vi "InstrChoice2.vi"(0 "Bras_OUT":bool, 5 "instruments.ini":path=path "C:/BonOMM_git/Config/instruments.ini") -> (6 "This VI's Path":path, 10 "Instrument Primaire OUT":string, 12 "Instrument Secondaire OUT":string, 14 "Instrument OUT":string, 15 "FoV 3":dbl caption="Champ de Vue" format="%.2g", 16 "foynom 3":i32 caption="Foyer nominale à 0°", 17 "atherm 3":dbl caption="Coefficient d'athermalisation" format="%.3g", 18 "exclusion 3":path caption="Chemin vers le fichier d'exclusion", 19 "collim 3":path caption="Chemin vers le fichier de collimation")   [LabVIEW 2019]
uses:
  <vilib>/Utility/config.llb/Read Key (String).vi
  <vilib>/Utility/config.llb/Read Key (Double).vi
  <vilib>/Utility/config.llb/Read Key (I32).vi
  <vilib>/Utility/config.llb/Read Key (Path).vi
  <vilib>/Utility/config.llb/Write Key (String).vi
  <vilib>/Utility/config.llb/Write Key (Boolean).vi
  <vilib>/Utility/config.llb/NI_LVConfig.lvlib
panel:
  out "Bool_primaire":bool
  out "Bool-Secondaire":bool
  out "Instrument Secondaire  IN":string
  out "Instrument Primaire  IN":string
  out "collim 2":path caption="Chemin vers le fichier de collimation"
  out "exclusion 2":path caption="Chemin vers le fichier d'exclusion"
  out "atherm 2":dbl caption="Coefficient d'athermalisation" format="%.3g"
  out "foynom 2":i32 caption="Foyer nominale à 0°"
  out "FoV 2":dbl caption="Champ de Vue" format="%.2g"
  in  "Instrument secondaire":i32(ring) items=["Pesto", "POMM", "CPAPIR", "Simon", "Spectro", "SpiOMM", "PANO-II+CCD4Kx4K", "CCD4Kx4K", "PANO-I+EMCCD", "POLARIMETRE"]
  out "collim":path caption="Chemin vers le fichier de collimation"
  out "exclusion":path caption="Chemin vers le fichier d'exclusion"
  out "FoV":dbl caption="Champ de Vue" format="%.2g"
  out "atherm":dbl caption="Coefficient d'athermalisation" format="%.3g"
  out "foynom":i32 caption="Foyer nominale à 0°"
  in  "ok":bool
  in  "Instruments primaire":i32(ring) items=["Pesto", "POMM", "CPAPIR", "Simon", "Spectro", "SpiOMM", "PANO-II+CCD4Kx4K", "CCD4Kx4K", "PANO-I+EMCCD", "POLARIMETRE"]
  # "[minutes d'arc]"
  # "[minutes d'arc]"
  # "[ADU]"
  # "[ADU]"
  # "[ADU/°K]"
  # "[ADU/°K]"
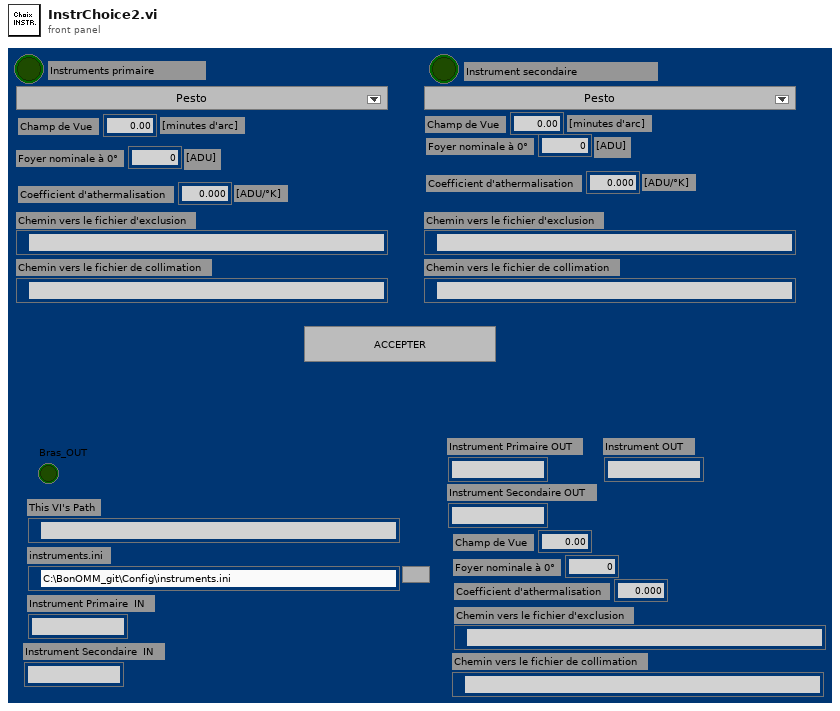
[diagram p1: front panel]
types:
  T1 = typedef "NI_LVConfig.lvlib/Config Data RefNum.ctl" = refnum<k1>
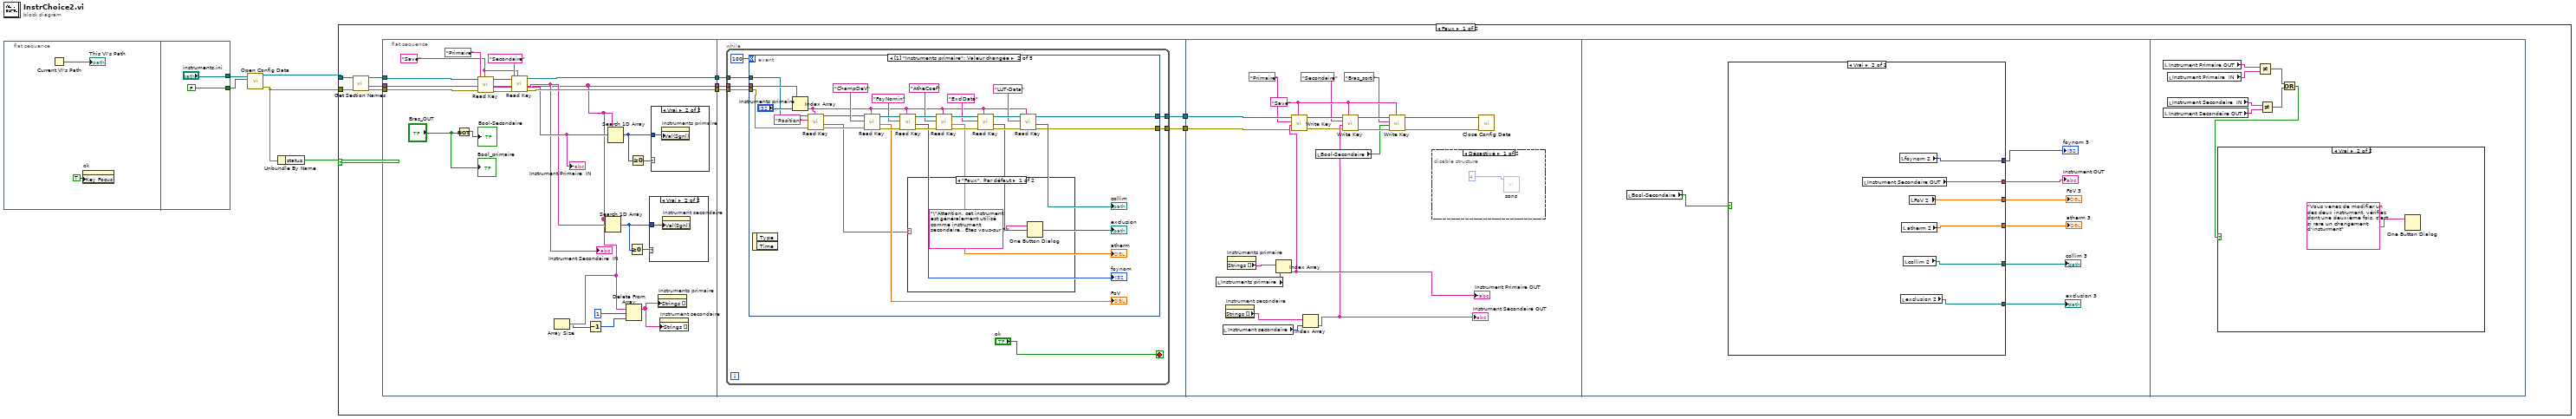
[diagram p0: block diagram]
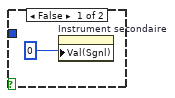
[diagram p2: hidden frame]
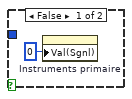
[diagram p3: hidden frame]
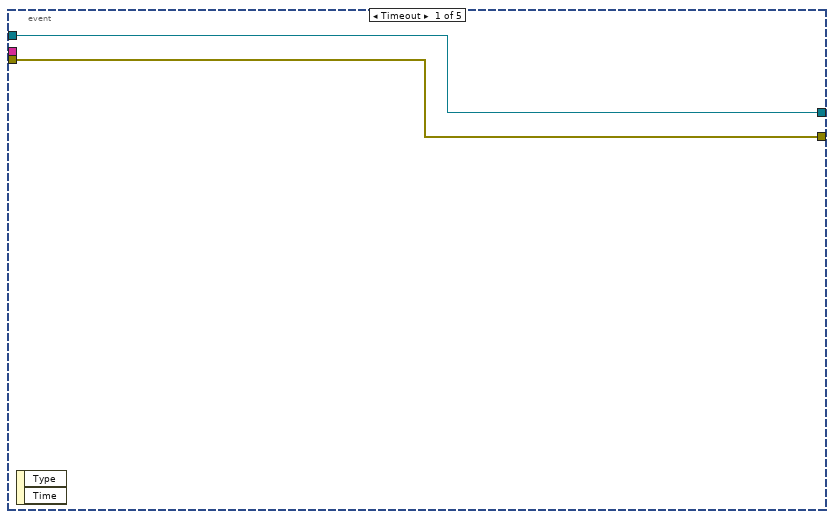
[diagram p4: hidden frame]
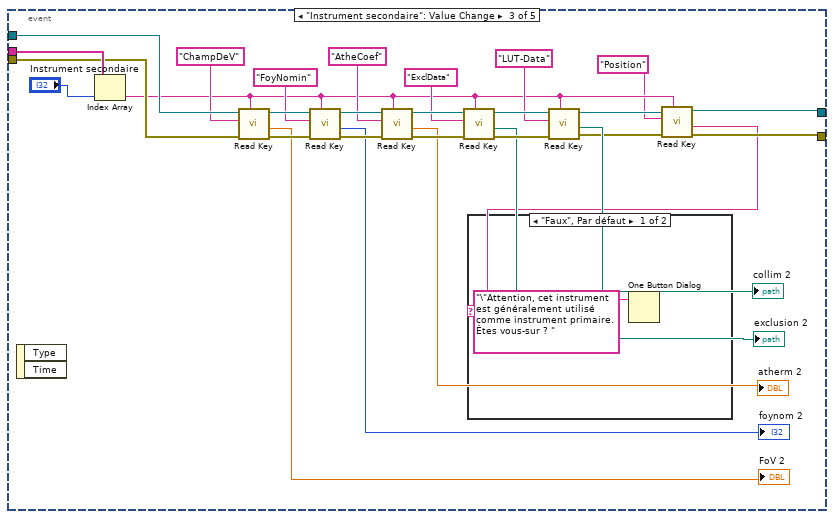
[diagram p6: hidden frame]
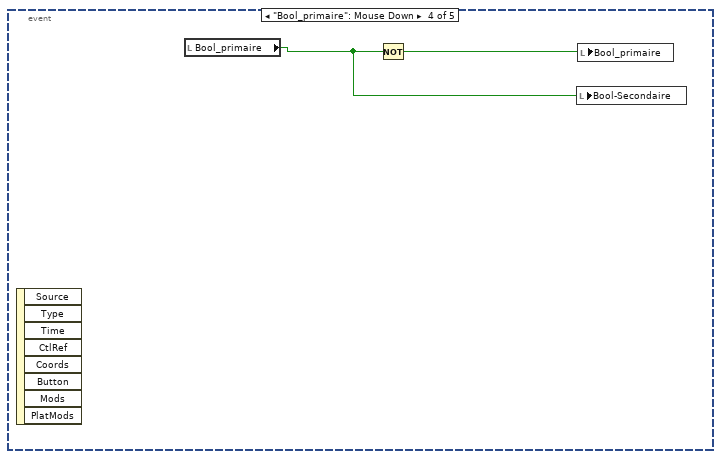
[diagram p8: hidden frame]
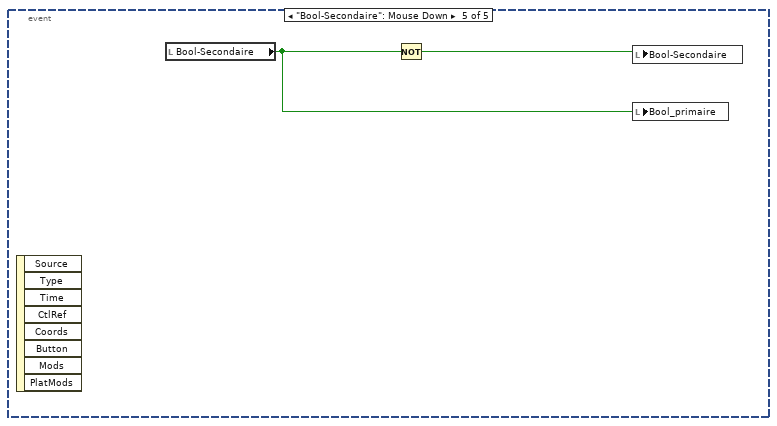
[diagram p9: hidden frame]
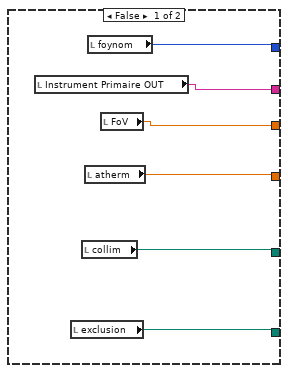
[diagram p11: hidden frame]
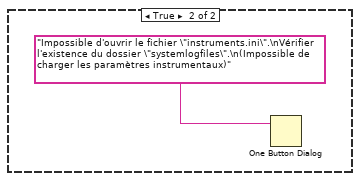
[diagram p13: hidden frame]
diagram:
  n1 = flat-sequence {
    tunnel: [FALSE ("create file if necessary (T)")] -> w5
    tunnel: ["instruments.ini"] -> w1
    frame #0 {
      n2 = Current VI's Path() -> (path=→"This VI's Path":path)
      n3 = property on="ok" class="Bool"("Key Focus"=TRUE) -> ()  [unwired: 2 in, 2 out]
    }
    frame #1 {
    }
  }
  n4 = call <vilib>:"Open Config Data.vi"("create file if necessary (T)"=w5, "configuration file path"=w1) -> ("error out"=w3:errorcluster, "refnum"=w4:T1)  [unwired: 7 in, 1 out]
  n5 = Unbundle By Name(w3) -> ("status"=w2:bool)
  n6 = case shown="Faux" w2 {
    tunnel: w4 -> [w19 _]
    tunnel: w3 -> [w18 _]
    frame False {
      n7 = call <vilib>:"Get Section Names.vi"("error in (no error)"=w18, "refnum"=w19) -> ("error out"=w15:errorcluster, "section names"=w16:string[], "refnum out"=w17:T1)  [unwired: 7 in]
      n8 = flat-sequence {
        tunnel: w17 -> [w23]
        tunnel: w16 -> [w27]
        tunnel: [w34] -> w14
        tunnel: w15 -> [w22]
        tunnel: [w37] -> w13
        tunnel: [w27] -> w12
        tunnel: w14 -> [w48]
        tunnel: w13 -> [w49]
        tunnel: w12 -> [w50]
        tunnel: [w47] -> w11
        tunnel: [w46] -> w10
        tunnel: w11 -> [w141]
        tunnel: w10 -> [w140]
        frame #0 {
          w24 = "Save" ("section")
          n9 = Not(x="Bras_OUT") -> (.not. x?=→"Bool-Secondaire":bool)
          n10 = call-poly <vilib>:"Read Key.vi"("section"=w24, "error in (no error)"=w22, "key"="Primaire", "refnum"=w23) -> ("error out"=w35:errorcluster, "value"=w33:string, "refnum out"=w38:T1)  [unwired: 4 in, 1 out]
          "Instrument Primaire  IN" <- w33
          n11 = call-poly <vilib>:"Read Key.vi"("section"=w24, "error in (no error)"=w35, "key"="Secondaire", "refnum"=w38) -> ("error out"=w34:errorcluster, "value"=w30:string, "refnum out"=w37:T1)  [unwired: 4 in, 1 out]
          "Instrument Secondaire  IN" <- w30
          n12 = Array Size(array=w27) -> (size(s)=w25:i32)
          n13 = Decrement(x=w25) -> (x-1=w26:i32)
          n14 = Search 1D Array(1D array=w27, element=w30) -> (index of element=w31:i32)  [unwired: 1 in]
          n15 = Search 1D Array(1D array=w27, element=w33) -> (index of element=w40:i32)  [unwired: 1 in]
          n16 = Delete From Array(array=w27, length=1 ("longueur"), index=w26) -> (array with subset deleted=w28:string[])  [unwired: 1 out]
          n17 = Greater Or Equal To 0?(x=w31) -> (x >= 0?=w32:bool)
          n18 = Greater Or Equal To 0?(x=w40) -> (x >= 0?=w41:bool)
          n19 = case shown="Vrai" w32 {
            tunnel: w31 -> [_ w43]
            frame False {
              n20 = property on="Instrument secondaire" class="MDér (strict)"("Val(Sgnl)"=0) -> ()  [unwired: 2 in, 2 out]
            }
            frame True {
              n21 = property on="Instrument secondaire" class="MDér (strict)"("Val(Sgnl)"=w43) -> ()  [unwired: 2 in, 2 out]
            }
          }
          n22 = case shown="Vrai" w41 {
            tunnel: w40 -> [_ w45]
            frame False {
              n23 = property on="Instruments primaire" class="MDér (strict)"("Val(Sgnl)"=0) -> ()  [unwired: 2 in, 2 out]
            }
            frame True {
              n24 = property on="Instruments primaire" class="MDér (strict)"("Val(Sgnl)"=w45) -> ()  [unwired: 2 in, 2 out]
            }
          }
          n25 = property on="Instruments primaire" class="MDér (strict)"("Strings []"=w28) -> ()  [unwired: 2 in, 2 out]
          n26 = property on="Instrument secondaire" class="MDér (strict)"("Strings []"=w28) -> ()  [unwired: 2 in, 2 out]
          "Bool_primaire" <- "Bras_OUT"
        }
        frame #1 {
          n27 = while {
            tunnel: w50 -> [w57]
            tunnel: w49 -> [w56]
            tunnel: w48 -> [w55]
            tunnel: [w53] -> w47
            tunnel: [w52] -> w46
            stop <- "ok" stop-if-true
            n28 = event shown="[1] \"Instruments primaire\": Valeur changée" {
              selector: _ -> [_ _ _ _ _]
              dyn-events: _ -> [_ _ _ _ _]
              timeout: 100 ("milliseconds to wait") -> [_ _ _ _ _]
              tunnel: w57 -> [_ w87 w118 _ _]
              tunnel: w56 -> [w59 w63 w117 _ _]
              tunnel: w55 -> [w58 w62 w116 _ _]
              tunnel: [w59 w68 w93 _ _] -> w53
              tunnel: [w58 w67 w94 _ _] -> w52
              event Timeout {
                n29 = event-data() -> ()  [unwired: 1 in, 2 out]
              }
              event "Instruments primaire": Value Change {
                n30 = event-data() -> ()  [unwired: 1 in, 2 out]
                n31 = Index Array(array=w87, index="Instruments primaire") -> (element=w65:string)
                n32 = call-poly <vilib>:"Read Key.vi"("section"=w65, "error in (no error)"=w62, "key"="Position", "refnum"=w63) -> ("error out"=w64:errorcluster, "value"=w60:string, "refnum out"=w66:T1)  [unwired: 4 in, 1 out]
                n33 = call-poly <vilib>:"Read Key.vi"("section"=w65, "error in (no error)"=w64, "key"="ChampDeV", "refnum"=w66) -> ("error out"=w85:errorcluster, "value"=→"FoV":dbl, "refnum out"=w86:T1)  [unwired: 4 in, 1 out]
                n34 = call-poly <vilib>:"Read Key.vi"("section"=w65, "error in (no error)"=w85, "key"="FoyNomin", "refnum"=w86) -> ("error out"=w83:errorcluster, "value"=→"foynom":i32, "refnum out"=w84:T1)  [unwired: 4 in, 1 out]
                n35 = case shown="\"Faux\", Par défaut" w60 {
                  frame "Faux", Default {
                    n36 = One Button Dialog(message="\"Attention, cet instrument est généralement utilisé comme instrument secondaire,. Êtes vous-sur ? ") -> ()  [unwired: 1 in, 1 out]
                  }
                  frame "Primaire" {
                  }
                }
                n37 = call-poly <vilib>:"Read Key.vi"("section"=w65, "error in (no error)"=w83, "key"="AtheCoef", "refnum"=w84) -> ("error out"=w79:errorcluster, "value"=→"atherm":dbl, "refnum out"=w80:T1)  [unwired: 4 in, 1 out]
                n38 = call-poly <vilib>:"Read Key.vi"("section"=w65, "error in (no error)"=w79, "key"="ExclData", "refnum"=w80) -> ("error out"=w82:errorcluster, "value"=→"exclusion":path, "refnum out"=w81:T1)  [unwired: 4 in, 1 out]
                n39 = call-poly <vilib>:"Read Key.vi"("section"=w65, "error in (no error)"=w82, "key"="LUT-Data", "refnum"=w81) -> ("error out"=w67:errorcluster, "value"=→"collim":path, "refnum out"=w68:T1)  [unwired: 4 in, 1 out]
              }
              event "Instrument secondaire": Value Change {
                n40 = event-data() -> ()  [unwired: 1 in, 2 out]
                n41 = Index Array(array=w118, index="Instrument secondaire") -> (element=w92:string)
                n42 = call-poly <vilib>:"Read Key.vi"("section"=w92, "error in (no error)"=w116, "key"="ChampDeV", "refnum"=w117) -> ("error out"=w114:errorcluster, "value"=→"FoV 2":dbl, "refnum out"=w115:T1)  [unwired: 4 in, 1 out]
                n43 = call-poly <vilib>:"Read Key.vi"("section"=w92, "error in (no error)"=w114, "key"="FoyNomin", "refnum"=w115) -> ("error out"=w112:errorcluster, "value"=→"foynom 2":i32, "refnum out"=w113:T1)  [unwired: 4 in, 1 out]
                n44 = call-poly <vilib>:"Read Key.vi"("section"=w92, "error in (no error)"=w112, "key"="AtheCoef", "refnum"=w113) -> ("error out"=w108:errorcluster, "value"=→"atherm 2":dbl, "refnum out"=w109:T1)  [unwired: 4 in, 1 out]
                n45 = call-poly <vilib>:"Read Key.vi"("section"=w92, "error in (no error)"=w108, "key"="ExclData", "refnum"=w109) -> ("error out"=w111:errorcluster, "value"=→"exclusion 2":path, "refnum out"=w110:T1)  [unwired: 4 in, 1 out]
                n46 = call-poly <vilib>:"Read Key.vi"("section"=w92, "error in (no error)"=w111, "key"="LUT-Data", "refnum"=w110) -> ("error out"=w95:errorcluster, "value"=→"collim 2":path, "refnum out"=w96:T1)  [unwired: 4 in, 1 out]
                n47 = call-poly <vilib>:"Read Key.vi"("section"=w92, "error in (no error)"=w95, "key"="Position", "refnum"=w96) -> ("error out"=w94:errorcluster, "value"=w90:string, "refnum out"=w93:T1)  [unwired: 4 in, 1 out]
                n48 = case shown="\"Faux\", Par défaut" w90 {
                  frame "Faux", Default {
                    n49 = One Button Dialog(message="\"Attention, cet instrument est généralement utilisé comme instrument primaire. Êtes vous-sur ? ") -> ()  [unwired: 1 in, 1 out]
                  }
                  frame "Secondaire" {
                  }
                }
              }
              event "Bool_primaire": Mouse Down {
                n50 = event-data() -> ()  [unwired: 1 in, 8 out]
                n51 = local read "Bool_primaire"() -> (w121:bool)
                n52 = Not(x=w121) -> (.not. x?=w120:bool)
                n53 = local write "Bool-Secondaire"(w121) -> ()
                n54 = local write "Bool_primaire"(w120) -> ()
              }
              event "Bool-Secondaire": Mouse Down {
                n55 = event-data() -> ()  [unwired: 1 in, 8 out]
                n56 = local read "Bool-Secondaire"() -> (w123:bool)
                n57 = Not(x=w123) -> (.not. x?=w122:bool)
                n58 = local write "Bool-Secondaire"(w122) -> ()
                n59 = local write "Bool_primaire"(w123) -> ()
              }
            }
          }
        }
        frame #2 {
          w128 = "Save" ("section")
          n60 = local read "Instruments primaire"() -> (w136:i32)
          n61 = local read "Instrument secondaire"() -> (w133:i32)
          n62 = property on="Instrument secondaire" class="MDér (strict)"() -> ("Strings []"=w134:string[])  [unwired: 2 in, 2 out]
          n63 = property on="Instruments primaire" class="MDér (strict)"() -> ("Strings []"=w135:string[])  [unwired: 2 in, 2 out]
          n64 = Index Array(array=w135, index=w136) -> (element=w142:string)
          "Instrument Primaire OUT" <- w142
          n65 = call-poly <vilib>:"Write Key.vi"("section"=w128, "error in (no error)"=w140, "value"=w142, "key"="Primaire", "refnum"=w141) -> ("error out"=w130:errorcluster, "refnum out"=w129:T1)  [unwired: 4 in, 1 out]
          n66 = Index Array(array=w134, index=w133) -> (element=w137:string)
          "Instrument Secondaire OUT" <- w137
          n67 = local read "Bool-Secondaire"() -> (w124:bool)
          n68 = call-poly <vilib>:"Write Key.vi"("section"=w128, "error in (no error)"=w130, "value"=w137, "key"="Secondaire", "refnum"=w129) -> ("error out"=w131:errorcluster, "refnum out"=w132:T1)  [unwired: 4 in, 1 out]
          n69 = call-poly <vilib>:"Write Key.vi"("section"=w128, "error in (no error)"=w131, "value"=w124, "key"="Bras_sorti", "refnum"=w132) -> ("error out"=w138:errorcluster, "refnum out"=w139:T1)  [unwired: 4 in, 1 out]
          n70 = disable-structure shown="Désactivé" {
            frame Disabled {
              n71 = call "sons.vi"("Index Son"=i16 4) -> ()  [unwired: 11 in]
            }
            frame Enabled {
            }
          }
          n72 = call <vilib>:"Close Config Data.vi"("error in (no error)"=w138, "refnum"=w139) -> ()  [unwired: 8 in, 2 out]
        }
        frame #3 {
          n73 = local read "Bool-Secondaire"() -> (w150:bool)
          n74 = case shown="Vrai" w150 {
            tunnel: [w156 w162] -> w147
            tunnel: [w155 w161] -> w149
            tunnel: [w154 w160] -> w146
            tunnel: [w153 w159] -> w144
            tunnel: [w152 w158] -> w145
            tunnel: [w151 w157] -> w148
            frame False {
              n75 = local read "Instrument Primaire OUT"() -> (w151:string)
              n76 = local read "exclusion"() -> (w153:path)
              n77 = local read "collim"() -> (w152:path)
              n78 = local read "atherm"() -> (w154:dbl)
              n79 = local read "foynom"() -> (w155:i32)
              n80 = local read "FoV"() -> (w156:dbl)
            }
            frame True {
              n81 = local read "Instrument Secondaire OUT"() -> (w157:string)
              n82 = local read "foynom 2"() -> (w161:i32)
              n83 = local read "exclusion 2"() -> (w159:path)
              n84 = local read "atherm 2"() -> (w160:dbl)
              n85 = local read "collim 2"() -> (w158:path)
              n86 = local read "FoV 2"() -> (w162:dbl)
            }
          }
          "FoV 3" <- w147
          "foynom 3" <- w149
          "exclusion 3" <- w144
          "atherm 3" <- w146
          "collim 3" <- w145
          "Instrument OUT" <- w148
        }
        frame #4 {
          n87 = local read "Instrument Primaire OUT"() -> (w169:string)
          n88 = local read "Instrument Secondaire OUT"() -> (w166:string)
          n89 = local read "Instrument Primaire  IN"() -> (w168:string)
          n90 = local read "Instrument Secondaire  IN"() -> (w167:string)
          n91 = Not Equal?(x=w169, y=w168) -> (x != y?=w165:bool)
          n92 = Not Equal?(x=w167, y=w166) -> (x != y?=w164:bool)
          n93 = Or(x=w165, y=w164) -> (x .or. y?=w163:bool)
          n94 = case shown="Vrai" w163 {
            frame False {
            }
            frame True {
              n95 = One Button Dialog(message="Vous venez de modifier un des deux instrument, vérifiez dont une deuxième fois, c'est si rare un changement d'insturment") -> ()  [unwired: 1 in, 1 out]
            }
          }
        }
      }
    }
    frame True {
      n96 = One Button Dialog(message="Impossible d'ouvrir le fichier \"instruments.ini\".\nVérifier l'existence du dossier \"systemlogfiles\".\n(Impossible de charger les paramètres instrumentaux)") -> ()  [unwired: 1 in, 1 out]
    }
  }
